vi "Rectangel GetRectInfo.vi"(2 "bounds":T1 {"height" format="%.2f"; "width" format="%.2f"; "y" format="%.2f"; "x" format="%.2f"}, 5 "error in (no error)":errorcluster) -> (15 "centerX":dbl format="%.2f", 16 "centerY":dbl format="%.2f", 17 "maxX":dbl format="%.2f", 18 "maxY":dbl format="%.2f", 19 "error out":errorcluster)   [LabVIEW 2016]
doc: "contains"
uses:
  <resource>/Framework/Providers/Open_GDS/UML/General/Rectangle/Rectangle Rectangle2D.ctl
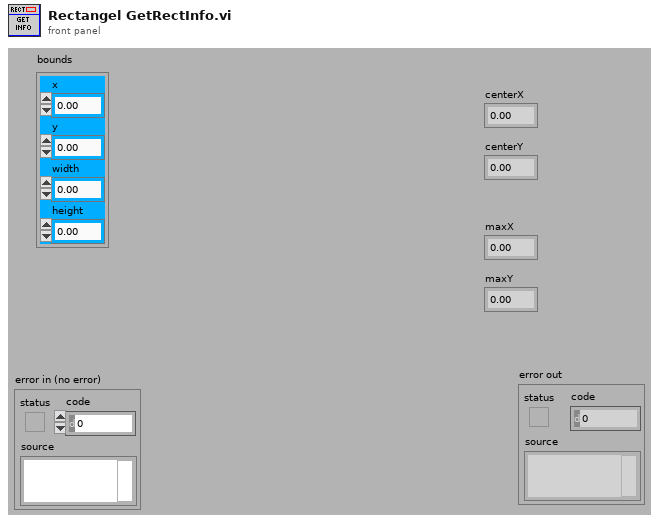
[diagram p1: front panel]
types:
  T1 = typedef "Rectangle Rectangle2D.ctl" = cluster{"x":dbl, "y":dbl, "width":dbl, "height":dbl}
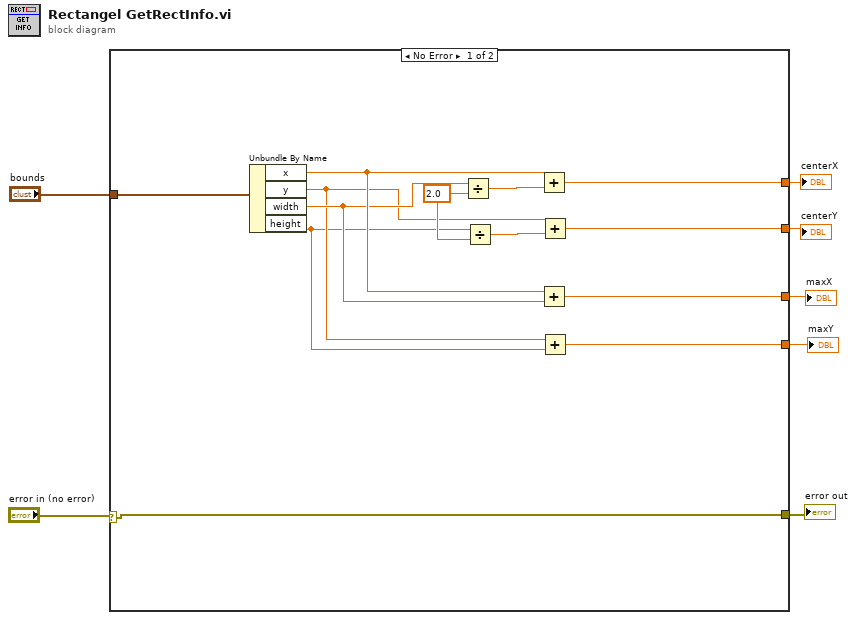
[diagram p0: block diagram]
diagram:
  n1 = case shown="No Error" "error in (no error)" {
    selector: "error in (no error)" -> [w19 w21]
    tunnel: [w19 w21] -> w7
    tunnel: "bounds" -> [w20 _]
    tunnel: [w15 _] -> w4
    tunnel: [w14 _] -> w3
    tunnel: [w9 _] -> w2
    tunnel: [w8 _] -> w1
    frame No Error {
      w16 = 2.0 ("y")
      n2 = Unbundle By Name(w20) -> ("x"=w13:dbl, "y"=w11:dbl, "width"=w12:dbl, "height"=w10:dbl)
      n3 = Divide(x=w12, y=w16) -> (x/y=w18:dbl)
      n4 = Divide(x=w10, y=w16) -> (x/y=w17:dbl)
      n5 = Add(x=w13, y=w18) -> (x+y=w15:dbl)
      n6 = Add(x=w13, y=w12) -> (x+y=w9:dbl)
      n7 = Add(x=w11, y=w17) -> (x+y=w14:dbl)
      n8 = Add(x=w11, y=w10) -> (x+y=w8:dbl)
    }
    frame Error {
    }
  }
  "error out" <- w7
  "centerY" <- w3
  "centerX" <- w4
  "maxX" <- w2
  "maxY" <- w1
